vi "MicroPulse - string to byte array + hdr.vi"(0 "SDO msg (hex)":string) -> (2 "header":u8 format="%.0x", 3 "[U8]":u8[](array[numeric]))   [LabVIEW 2026, in "MicroPulse_Driver.lvlib"]
uses:
  MicroPulse_Driver.lvlib
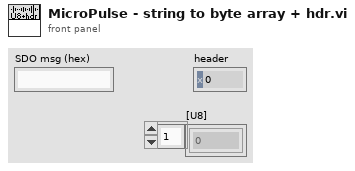
[diagram p1: front panel]
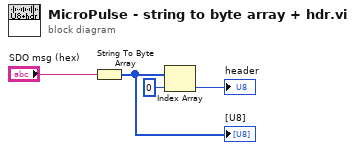
[diagram p0: block diagram]
diagram:
  n1 = String To Byte Array(string="SDO msg (hex)") -> (unsigned byte array=w4:u8[])
  "[U8]" <- w4
  n2 = Index Array(array=w4, index=0) -> (element=→"header":u8)
